vi "_102.vi"() -> ()   [LabVIEW 2020]
panel:
  out "String":string
  out "Boolean":bool
  out "x/y":dbl
  in  "Numeric":dbl
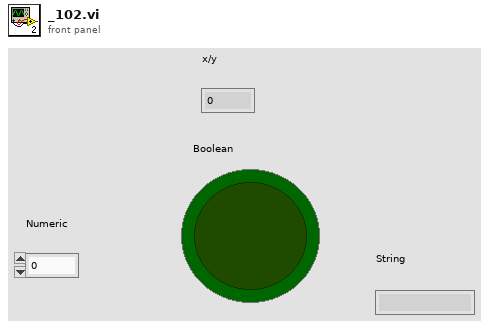
[diagram p1: front panel]
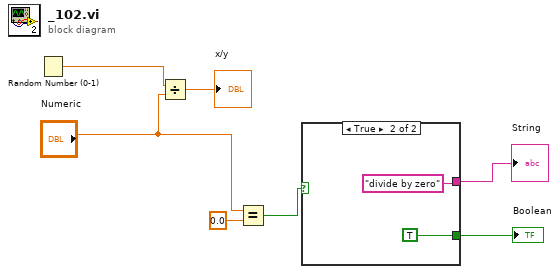
[diagram p0: block diagram]
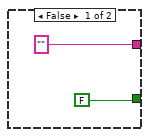
[diagram p2: hidden frame]
diagram:
  n1 = Random Number (0-1)() -> (number: 0 to 1=w7:dbl)
  n2 = Divide(x=w7, y="Numeric") -> (x/y=→"x/y":dbl)
  n3 = Equal?(x="Numeric", y=0.0) -> (x = y?=w2:bool)
  n4 = case shown="True" w2 {
    tunnel: [FALSE TRUE] -> w5
    tunnel: ["" "divide by zero"] -> w1
    frame False {
    }
    frame True {
    }
  }
  "Boolean" <- w5
  "String" <- w1
